vi "Select Color.vi"(10 "Color":T1=30 items=["Black"=30, "Red"=31, "Green"=32, "Yellow"=33, "Blue"=34, "Magenta"=35, "Cyan"=36, "White"=37, "Gray"=90, "Bright Red"=91, "Bright Green"=92, "Bright Yellow"=93, "Bright Blue"=94, "Bright Magenta"=95, "Bright Cyan"=96, "Bright White"=97], 11 "Color Scheme":T2={"Black"=2302755, "Red"=16711695, "Green"=9232651, "Yellow"=16759040, "Blue"=36344, "Magenta"=7160742, "Cyan"=55531, "White"=15132390, "Bright Black"=4473924, "Bright Red"=16721728, "Bright Green"=11264347, "Bright Yellow"=16765506, "Bright Blue"=37631, "Bright Magenta"=10117099, "Bright Cyan"=6815728, "Bright White"=16777215}) -> (3 "Color Value":u32(colorbox))   [LabVIEW 2020, in "Terminal.lvlib" / "Terminal.lvclass"]
uses:
  Terminal.lvclass
  Terminal.lvclass/Terminal.ctl
  Color Scheme.ctl
  Terminal.lvlib
  Color.ctl
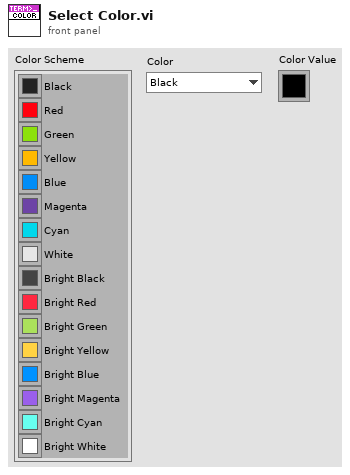
[diagram p1: front panel]
types:
  T1 = typedef "Terminal.lvlib/Color.ctl" = i8
  T2 = typedef "Terminal.lvlib/Color Scheme.ctl" = cluster{"Black":u32, "Red":u32, "Green":u32, "Yellow":u32, "Blue":u32, "Magenta":u32, "Cyan":u32, "White":u32, "Bright Black":u32, "Bright Red":u32, "Bright Green":u32, "Bright Yellow":u32, "Bright Blue":u32, "Bright Magenta":u32, "Bright Cyan":u32, "Bright White":u32}
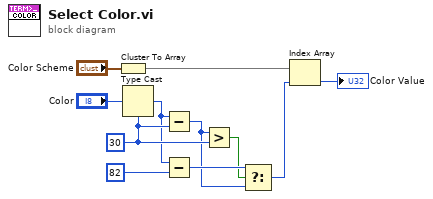
[diagram p0: block diagram]
diagram:
  w10 = i8 30
  n1 = Cluster To Array(cluster="Color Scheme") -> (array=w3:u32[])
  n2 = Type Cast(type=w10, x="Color") -> (*(type *) &x=w9:i8)
  n3 = Subtract(x=w9, y=w10) -> (x-y=w5:i8)
  n4 = Subtract(x=w9, y=i8 82) -> (x-y=w7:i8)
  n5 = Greater?(x=w5, y=w10) -> (0:w6:bool)
  n6 = Select(t=w7, s=w6, f=w5) -> (s? t:f=w2:i8)
  n7 = Index Array(array=w3, index=w2) -> (element=→"Color Value":u32)
